vi "Take Outline Image.vi"(5 "Outline Width":dbl, 6 "Image Name":string="composite image", 7 "Quality":enum16{"perfect", "high", "medium", "low"}(ring), 8 "error in (no error)":errorcluster, 9 "Field of View":cluster{"Size-X(mm)":dbl, "Size-Y(mm)":dbl}, 10 "Image Center":refnum<class "Vec3d.lvclass">, 11 "Gantry in":refnum<class "Gantry.lvclass">) -> (0 "error out":errorcluster, 3 "Gantry out":refnum<class "Gantry.lvclass">)   [LabVIEW 2023, in "Gantry.lvclass"]
uses:
  Gantry.lvclass
  Vec3d Class/Vec3d.lvclass
  Utils/Type Definitions/Physical Image.ctl
  <vilib>/vision/Image Controls.llb/IMAQ Image.ctl
panel:
  out "Physical Image":T1
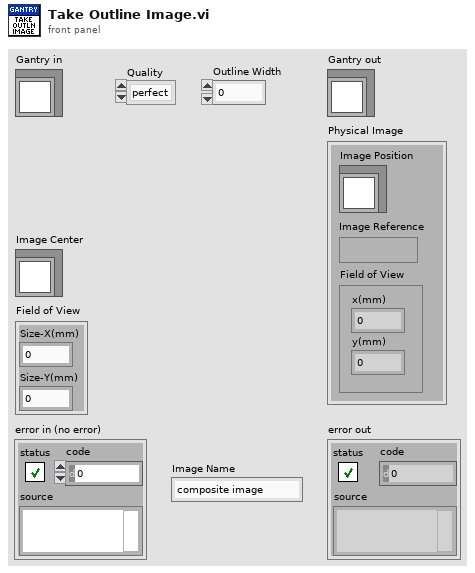
[diagram p1: front panel]
types:
  T1 = typedef "Physical Image.ctl" = cluster{"Image Position":refnum<class "Vec3d.lvclass">, "Image Reference":T2, "Field of View":cluster{"x(mm)":dbl, "y(mm)":dbl}}
  T2 = typedef "IMAQ Image.ctl" = refnum<image>
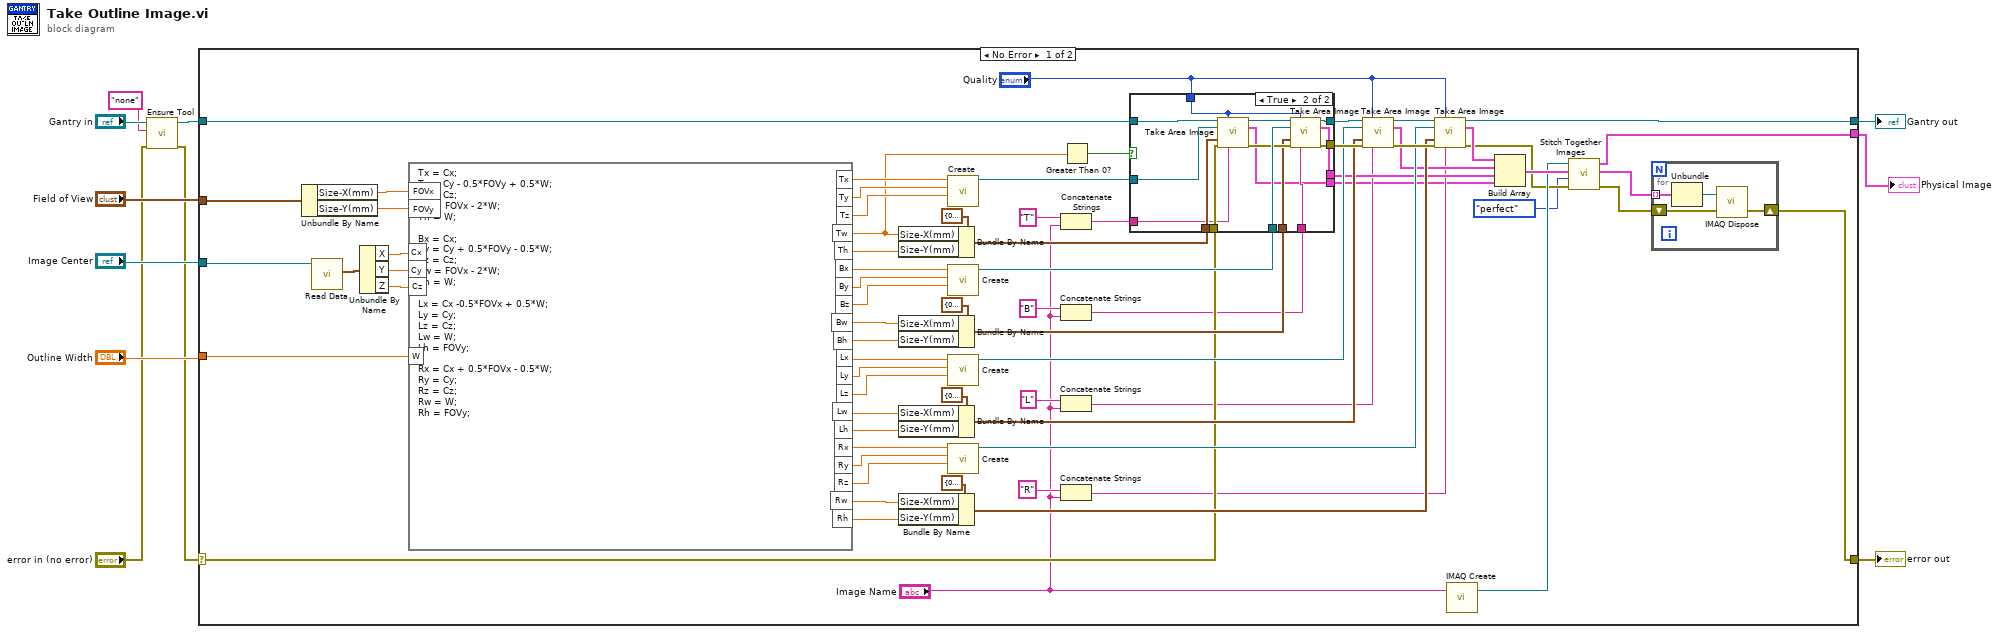
[diagram p0: block diagram]
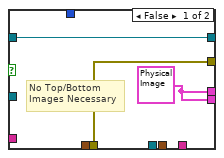
[diagram p2: hidden frame]
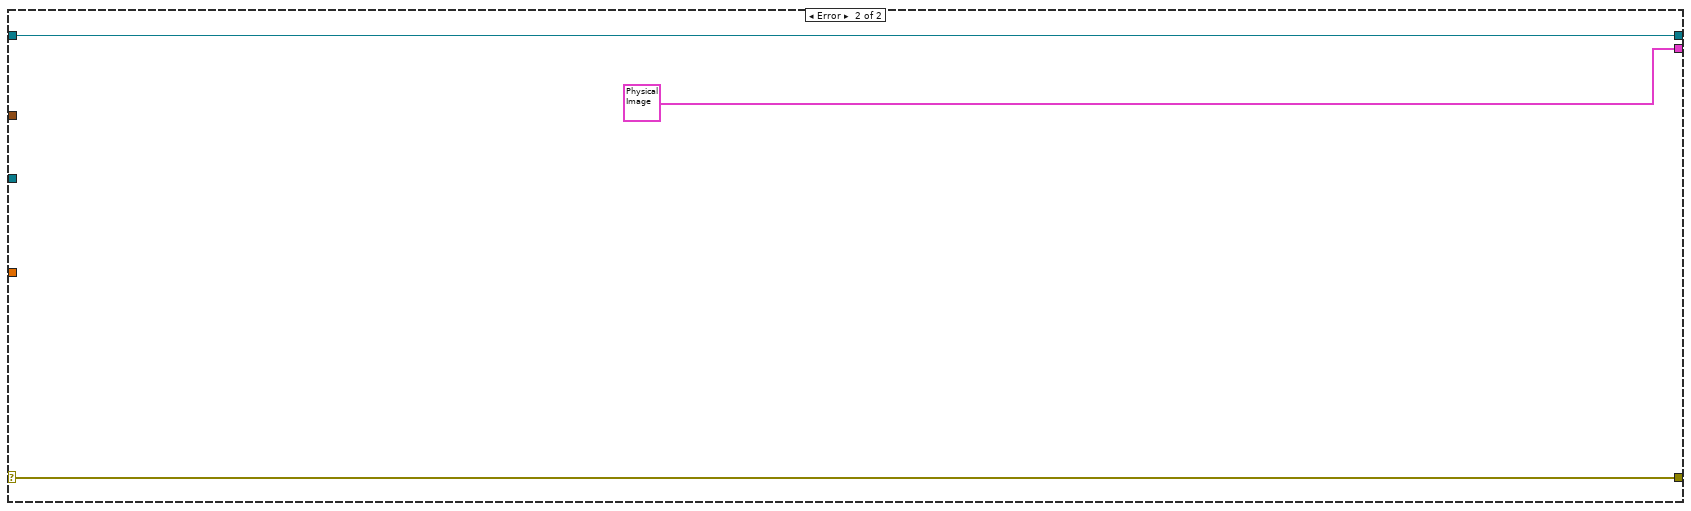
[diagram p3: hidden frame]
diagram:
  n1 = call "Ensure Tool.vi"("error in (no error)"="error in (no error)", "Tool Name"="none", "Gantry in"="Gantry in") -> ("error out"=w2:errorcluster, "Gantry out"=w4:refnum<class "Gantry.lvclass">)  [unwired: 7 in]
  n2 = case shown="No Error" w2 {
    selector: w2 -> [w36 w107]
    tunnel: [w18 w107] -> w6
    tunnel: [w47 w106] -> w7
    tunnel: w4 -> [w50 w106]
    tunnel: "Field of View" -> [w81 _]
    tunnel: "Image Center" -> [w82 _]
    tunnel: [w29 T1 {"Image Position"=refnum, "Image Reference"=refnum, "Field of View"={"x(mm)"=0.0, "y(mm)"=0.0}} ("Physical Image")] -> w8
    tunnel: "Outline Width" -> [w74 _]
    frame No Error {
      n3 = Unbundle By Name(w81) -> ("Size-X(mm)"=w80:dbl, "Size-Y(mm)"=w79:dbl)
      n4 = call-dynamic "Read Data.vi"("Vec3d Class in"=w82) -> ("Data"=w78:cluster{"X":dbl, "Y":dbl, "Z":dbl})  [unwired: 8 in, 2 out]
      n5 = Unbundle By Name(w78) -> ("X"=w77:dbl, "Y"=w76:dbl, "Z"=w75:dbl)
      n6 = formula code="Tx = Cx;\nTy = Cy - 0.5*FOVy + 0.5*W;\nTz = Cz;\nTw = FOVx - 2*W;\nTh = W;\n\nBx = Cx;\nBy = Cy + 0.5*FOVy - 0.5*W;\nBz = Cz;\nBw = FOVx - 2*W;\nBh = W;\n\nLx = Cx -0.5*FOVx + 0.5*W;\nLy = Cy;\nLz = Cz;\nLw = W;\nLh = FOVy;\n\nRx = Cx + 0.5*FOVx - 0.5*W;\nRy = Cy;\nRz = Cz;\nRw = W;\nRh = FOVy;"("Cx"=w77, "Cy"=w76, "Cz"=w75, "FOVx"=w80, "FOVy"=w79, "W"=w74) -> ("Tx"=w73:dbl, "Ty"=w72:dbl, "Tz"=w71:dbl, "Tw"=w16:dbl, "Th"=w69:dbl, "Bx"=w67:dbl, "By"=w66:dbl, "Bz"=w65:dbl, "Bw"=w64:dbl, "Bh"=w63:dbl, "Lx"=w61:dbl, "Ly"=w60:dbl, "Lz"=w59:dbl, "Lw"=w58:dbl, "Lh"=w57:dbl, "Rx"=w55:dbl, "Ry"=w54:dbl, "Rz"=w53:dbl, "Rw"=w52:dbl, "Rh"=w51:dbl)
      n7 = Bundle By Name(cluster=cluster{"Size-X(mm)":dbl, "Size-Y(mm)":dbl} {"Size-X(mm)"=0.0, "Size-Y(mm)"=0.0} ("Field of View"), "Size-X(mm)"=w16, "Size-Y(mm)"=w69) -> (w45:cluster{"Size-X(mm)":dbl, "Size-Y(mm)":dbl})
      n8 = Bundle By Name(cluster=cluster{"Size-X(mm)":dbl, "Size-Y(mm)":dbl} {"Size-X(mm)"=0.0, "Size-Y(mm)"=0.0} ("Field of View"), "Size-X(mm)"=w64, "Size-Y(mm)"=w63) -> (w41:cluster{"Size-X(mm)":dbl, "Size-Y(mm)":dbl})
      n9 = Bundle By Name(cluster=cluster{"Size-X(mm)":dbl, "Size-Y(mm)":dbl} {"Size-X(mm)"=0.0, "Size-Y(mm)"=0.0} ("Field of View"), "Size-X(mm)"=w58, "Size-Y(mm)"=w57) -> (w39:cluster{"Size-X(mm)":dbl, "Size-Y(mm)":dbl})
      n10 = Bundle By Name(cluster=cluster{"Size-X(mm)":dbl, "Size-Y(mm)":dbl} {"Size-X(mm)"=0.0, "Size-Y(mm)"=0.0} ("Field of View"), "Size-X(mm)"=w52, "Size-Y(mm)"=w51) -> (w37:cluster{"Size-X(mm)":dbl, "Size-Y(mm)":dbl})
      n11 = call "Create.vi"("Z"=w71, "Y"=w72, "X"=w73) -> ("Vec3d Class out"=w46:refnum<class "Vec3d.lvclass">)  [unwired: 7 in, 1 out]
      n12 = call "Create.vi"("Z"=w65, "Y"=w66, "X"=w67) -> ("Vec3d Class out"=w44:refnum<class "Vec3d.lvclass">)  [unwired: 7 in, 1 out]
      n13 = call "Create.vi"("Z"=w59, "Y"=w60, "X"=w61) -> ("Vec3d Class out"=w40:refnum<class "Vec3d.lvclass">)  [unwired: 7 in, 1 out]
      n14 = call "Create.vi"("Z"=w53, "Y"=w54, "X"=w55) -> ("Vec3d Class out"=w38:refnum<class "Vec3d.lvclass">)  [unwired: 7 in, 1 out]
      n15 = Concatenate Strings("T", "Image Name") -> (w27:string)
      n16 = Concatenate Strings("B", "Image Name") -> (w23:string)
      n17 = Concatenate Strings("L", "Image Name") -> (w22:string)
      n18 = Concatenate Strings("R", "Image Name") -> (w21:string)
      n19 = Greater Than 0?(x=w16) -> (x > 0?=w15:bool)
      n20 = case shown="True" w15 {
        tunnel: w50 -> [w89 w104]
        tunnel: [w89 w102] -> w49
        tunnel: "Quality" -> [_ w90]
        tunnel: w46 -> [_ w101]
        tunnel: w45 -> [_ w100]
        tunnel: w44 -> [_ w99]
        tunnel: [w87 w97] -> w43
        tunnel: w41 -> [_ w96]
        tunnel: w36 -> [w87 w95]
        tunnel: [w88 w94] -> w35
        tunnel: w27 -> [_ w93]
        tunnel: w23 -> [_ w92]
        tunnel: [w88 w91] -> w17
        frame False {
          w88 = T1 {"Image Position"=refnum, "Image Reference"=refnum, "Field of View"={"x(mm)"=0.0, "y(mm)"=0.0}} ("Physical Image")
          # "No Top/Bottom\nImages Necessary"
        }
        frame True {
          n21 = call "Take Area Image.vi"("Gantry in"=w104, "Quality"=w90, "Image Center"=w101, "Field of View"=w100, "error in (no error)"=w95, "Image Name"=w93) -> ("Gantry out"=w103:refnum<class "Gantry.lvclass">, "Physical Image"=w91:T1, "error out"=w98:errorcluster)  [unwired: 7 in]
          n22 = call "Take Area Image.vi"("Gantry in"=w103, "Quality"=w90, "Image Center"=w99, "Field of View"=w96, "error in (no error)"=w98, "Image Name"=w92) -> ("Gantry out"=w102:refnum<class "Gantry.lvclass">, "Physical Image"=w94:T1, "error out"=w97:errorcluster)  [unwired: 7 in]
        }
      }
      n23 = call "Take Area Image.vi"("Gantry in"=w49, "Quality"="Quality", "Image Center"=w40, "Field of View"=w39, "error in (no error)"=w43, "Image Name"=w22) -> ("Gantry out"=w48:refnum<class "Gantry.lvclass">, "Physical Image"=w34:T1, "error out"=w42:errorcluster)  [unwired: 7 in]
      n24 = call "Take Area Image.vi"("Gantry in"=w48, "Quality"="Quality", "Image Center"=w38, "Field of View"=w37, "error in (no error)"=w42, "Image Name"=w21) -> ("Gantry out"=w47:refnum<class "Gantry.lvclass">, "Physical Image"=w33:T1, "error out"=w30:errorcluster)  [unwired: 7 in]
      n25 = call "IMAQ Create"("Image Name"="Image Name") -> ("New Image"=w31:T2)  [unwired: 4 in, 1 out]
      n26 = Build Array(w33, w34, w35, w17) -> (w32:T1[])
      n27 = call "Stitch Together Images.vi"("error in"=w30, "Quality"=enum16{"perfect", "high", "medium", "low"}."perfect", "Physical Images in"=w32, "Image Dst"=w31) -> ("error out"=w19:errorcluster, "Physical Images out"=w20:T1[], "Composite Physical Image"=w29:T1)  [unwired: 5 in]
      n28 = for {
        tunnel: w20 -> [w86] mode=indexing
        shift-right: [w83] -> w18
        shift-left: w19 -> [w84]
        n29 = Unbundle(w86) -> ("Image Reference"=w85:T2)  [unwired: 2 out]
        n30 = call "IMAQ Dispose"("Image"=w85, "error in (no error)"=w84) -> ("error out"=w83:errorcluster)  [unwired: 4 in]
      }
    }
    frame Error {
    }
  }
  "error out" <- w6
  "Gantry out" <- w7
  "Physical Image" <- w8
